vi "Variant to Key List.vi"(5 "section":string, 7 "Prefix":string, 8 "Error In":errorcluster, 10 "Label.Text":string, 11 "Variant":variant) -> (0 "Error Out":errorcluster, 2 "Key list":T1)   [LabVIEW 2015]
uses:
  <vilib>/Utility/Data Type/NI_Data Type.lvlib
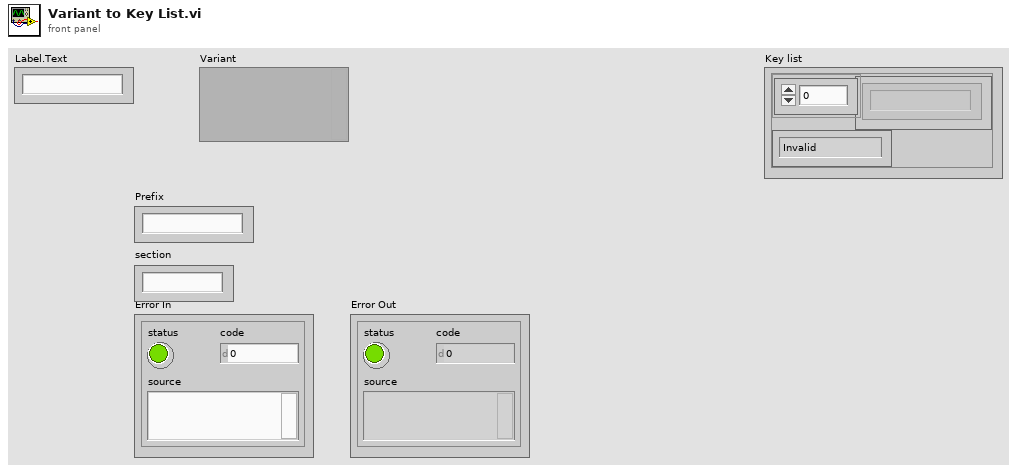
[diagram p1: front panel]
types:
  T1 = cluster{"Array":string[], "Enum":enum16{"Invalid", "Boolean", "Double", "I32", "Path", "String", "U32", "Array", "Cluster"}}
  T2 = typedef "NI_Data Type.lvlib/Data Type.ctl" = enum8{"Invalid Type", "Void", "I8", "I16", "I32", "I64", "U8", "U16", "U32", "U64", "Single Float", "Double Float", "Extended Float", "Single Complex", "Double Complex", "Extended Complex", "Enum U8", "Enum U16", "Enum U32", "Enum U64", "Single Float With Unit", "Double Float With Unit", "Extended Float With Unit", "Single Complex with Unit", "Double Complex with Unit", "Extended Complex with Unit", "Boolean", "String", "Path", "Picture", "Tag", "Array", "Cluster", "Variant", "LV Variant", "Waveform", "Timestamp", "Digital Waveform", "Digital Data", "ExpressData", "Refnum", "External Data", "VI", "Poly VI", "LabVIEW Class Instance", "Fixed Point"}
  T3 = enum16{"Invalid", "Boolean", "Double", "I32", "Path", "String", "U32", "Array", "Cluster"}
  T4 = cluster{string[], enum16{"Invalid", "Boolean", "Double", "I32", "Path", "String", "U32", "Array", "Cluster"}}
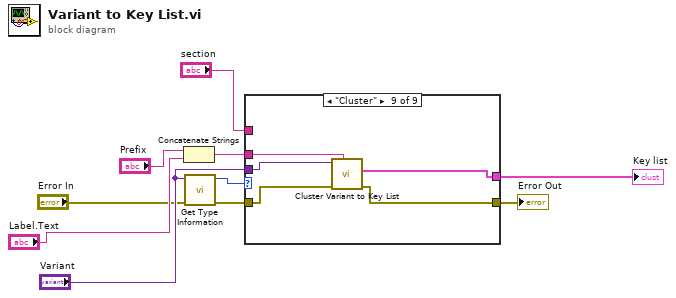
[diagram p0: block diagram]
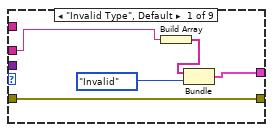
[diagram p2: hidden frame]
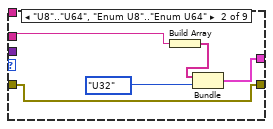
[diagram p3: hidden frame]
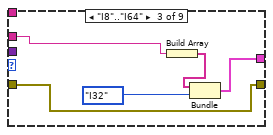
[diagram p4: hidden frame]
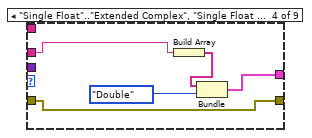
[diagram p5: hidden frame]
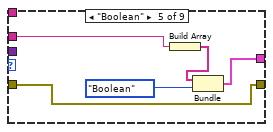
[diagram p6: hidden frame]
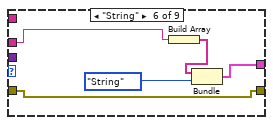
[diagram p7: hidden frame]
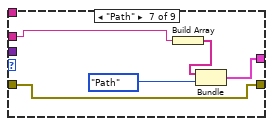
[diagram p8: hidden frame]
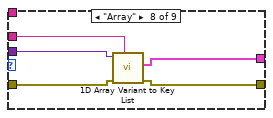
[diagram p9: hidden frame]
diagram:
  n1 = Concatenate Strings("Prefix", "Label.Text") -> (w7:string)
  n2 = call <vilib>:"Get Type Information.vi"("error in (no error)"="Error In", "Variant"="Variant") -> ("error out"=w6:errorcluster, "Type"=w10:T2)  [unwired: 5 in, 3 out]
  n3 = case shown="\"Cluster\"" w10 {
    tunnel: "section" -> [_ _ _ _ _ _ _ _ _]
    tunnel: w7 -> [w12 w18 w21 w26 w35 w37 w41 w47 w52]
    tunnel: w6 -> [w15 w16 w23 w28 w32 w38 w43 w50 w55]
    tunnel: [w15 w16 w23 w28 w32 w38 w43 w49 w54] -> w5
    tunnel: "Variant" -> [_ _ _ _ _ _ _ w48 w51]
    tunnel: [w11 w17 w22 w27 w31 w36 w42 w46 w53] -> w4
    frame "Invalid Type", Default {
      n4 = Build Array(w12) -> (w14:string[])
      n5 = Bundle(w14, T3."Invalid") -> (w11:T4)  [unwired: 1 in]
    }
    frame "U8".."U64", "Enum U8".."Enum U64" {
      n6 = Build Array(w18) -> (w20:string[])
      n7 = Bundle(w20, T3."U32") -> (w17:T4)  [unwired: 1 in]
    }
    frame "I8".."I64" {
      n8 = Build Array(w21) -> (w25:string[])
      n9 = Bundle(w25, T3."I32") -> (w22:T4)  [unwired: 1 in]
    }
    frame "Single Float".."Extended Complex", "Single Float With Unit".."Extended Complex with Unit" {
      n10 = Build Array(w26) -> (w30:string[])
      n11 = Bundle(w30, T3."Double") -> (w27:T4)  [unwired: 1 in]
    }
    frame "Boolean" {
      n12 = Build Array(w35) -> (w34:string[])
      n13 = Bundle(w34, T3."Boolean") -> (w31:T4)  [unwired: 1 in]
    }
    frame "String" {
      n14 = Build Array(w37) -> (w40:string[])
      n15 = Bundle(w40, T3."String") -> (w36:T4)  [unwired: 1 in]
    }
    frame "Path" {
      n16 = Build Array(w41) -> (w45:string[])
      n17 = Bundle(w45, T3."Path") -> (w42:T4)  [unwired: 1 in]
    }
    frame "Array" {
      n18 = call "1D Array Variant to Key List.vi"("Prefix"=w47, "Error In"=w50, "Variant"=w48) -> ("Error Out"=w49:errorcluster, "Key list"=w46:T1)  [unwired: 7 in]
    }
    frame "Cluster" {
      n19 = call "Cluster Variant to Key List.vi"("Prefix"=w52, "Error In"=w55, "Variant"=w51) -> ("Error Out"=w54:errorcluster, "Key list"=w53:T1)  [unwired: 7 in]
    }
  }
  "Error Out" <- w5
  "Key list" <- w4
